vi "Select 1010.vi"(2 "error in (no error)":errorcluster, 3 "Parameters Select":T1) -> (0 "error out":errorcluster, 1 "Array":bool[](array[boolean]))   [LabVIEW 2015]
uses:
  C1G2_CommandControl.ctl
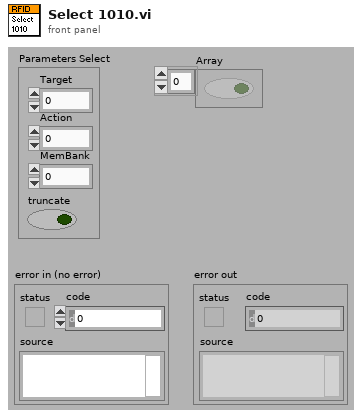
[diagram p1: front panel]
types:
  T1 = cluster{"Target":u16, "Action":u16, "MemBank":u16, "truncate":bool}
  T2 = typedef "C1G2_CommandControl.ctl" = u16
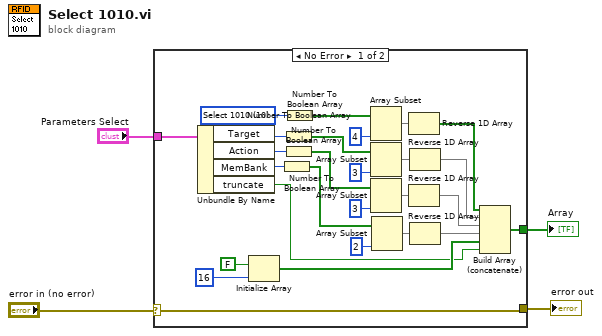
[diagram p0: block diagram]
diagram:
  n1 = case shown="No Error" "error in (no error)" {
    selector: "error in (no error)" -> [w5 w32]
    tunnel: [w31 _] -> w4
    tunnel: "Parameters Select" -> [w10 _]
    tunnel: [w5 w32] -> w1
    frame No Error {
      w6 = T2 10 items=["Select 1010"=10, "Query 1000"=8] ("Command")
      n2 = Unbundle By Name(w10) -> ("Target"=w7:u16, "Action"=w8:u16, "MemBank"=w9:u16, "truncate"=w11:bool)
      n3 = Initialize Array(FALSE, 16 ("dimension size")) -> (w26:bool[])
      n4 = Number To Boolean Array(number=w9) -> (Boolean array=w18:bool[])
      n5 = Number To Boolean Array(number=w7) -> (Boolean array=w16:bool[])
      n6 = Number To Boolean Array(number=w8) -> (Boolean array=w17:bool[])
      n7 = Number To Boolean Array(number=w6) -> (Boolean array=w14:bool[])
      n8 = Array Subset(array=w14, length=4) -> (w15:bool[])  [unwired: 1 in]
      n9 = Array Subset(array=w16, length=3) -> (w23:bool[])  [unwired: 1 in]
      n10 = Array Subset(array=w17, length=3) -> (w24:bool[])  [unwired: 1 in]
      n11 = Array Subset(array=w18, length=2) -> (w25:bool[])  [unwired: 1 in]
      n12 = Reverse 1D Array(array=w15) -> (reversed array=w27:bool[])
      n13 = Reverse 1D Array(array=w24) -> (reversed array=w29:bool[])
      n14 = Reverse 1D Array(array=w23) -> (reversed array=w28:bool[])
      n15 = Reverse 1D Array(array=w25) -> (reversed array=w30:bool[])
      n16 = Build Array (concatenate)(w27, w28, w29, w30, w26, w11) -> (w31:bool[])
    }
    frame Error {
    }
  }
  "Array" <- w4
  "error out" <- w1
